vi "兩陣列相加.vi"(5 "X原":dbl, 7 "Y原":dbl, 9 "INDEX":i32=2, 10 "++Y":dbl[](array[numeric])=[0.0], 11 "++X":dbl[](array[numeric])=[0.0]) -> (2 "Y array":dbl[](array[numeric]), 3 "X array":dbl[](array[numeric]))   [LabVIEW 2015]
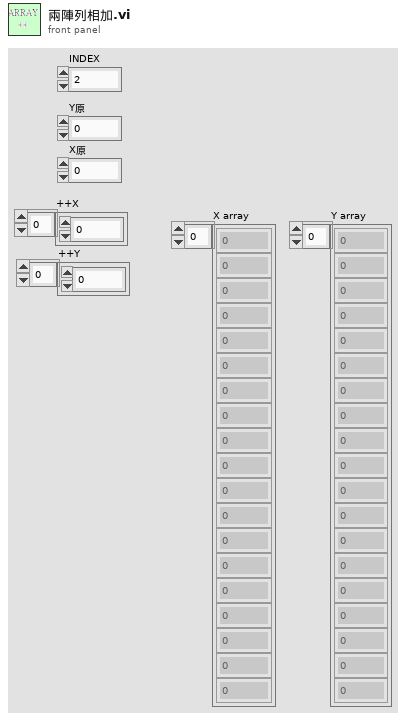
[diagram p1: front panel]
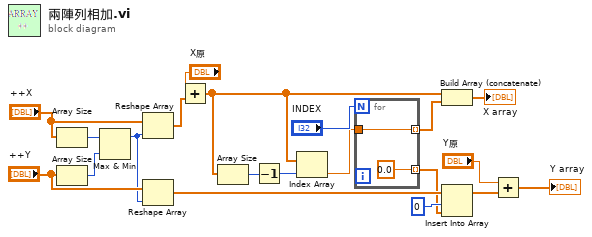
[diagram p0: block diagram]
diagram:
  n1 = Array Size(array="++X") -> (size(s)=w20:i32)
  n2 = Array Size(array="++Y") -> (size(s)=w19:i32)
  n3 = Max & Min(x=w20, y=w19) -> (max(x,y)=w10:i32)  [unwired: 1 out]
  n4 = Reshape Array("++X", w10) -> (w11:dbl[])
  n5 = Reshape Array("++Y", w10) -> (w15:dbl[])
  n6 = Add(x="X原", y=w11) -> (x+y=w4:dbl[])
  n7 = Array Size(array=w4) -> (size(s)=w5:i32)
  n8 = Decrement(x=w5) -> (x-1=w7:i32)
  n9 = Index Array(array=w4, index=w7) -> (element=w2:dbl)
  n10 = for {
    N: "INDEX" -> [_]
    tunnel: [0.0] -> w14 mode=indexing
    tunnel: [w21] -> w1 mode=indexing
    tunnel: w2 -> [w21]
  }
  n11 = Build Array (concatenate)(w4, w1) -> (→"X array":dbl[])
  n12 = Insert Into Array(array=w15, index=0, new element=w14) -> (w12:dbl[])
  n13 = Add(x="Y原", y=w12) -> (x+y=→"Y array":dbl[])
